vi "swingup_energy_controller.vi"(1 "mu (m/s^2/J)":dbl, 2 "max_u (m/s^2)":dbl=5.0, 3 "alpha_dot (rad/s)":dbl, 4 "alpha_full (rad)":dbl, 5 "E (mJ)":dbl, 6 "Er (mJ)":dbl) -> (0 "u (m/s^2)":dbl)   [LabVIEW 2010]
doc: "Calculates the desired linear acceleration of the pendulum pivot required to swing the pendulum towards the upright position."
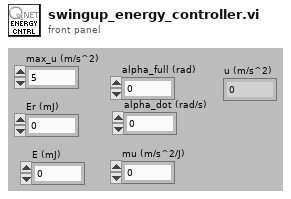
[diagram p1: front panel]
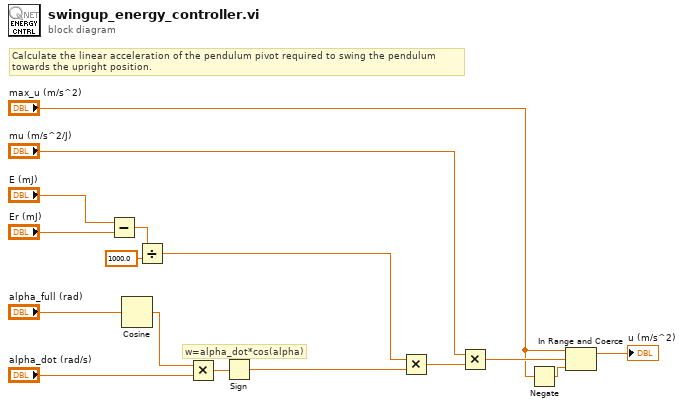
[diagram p0: block diagram]
diagram:
  # "w=alpha_dot*cos(alpha)"
  # "Calculate the linear acceleration of the pendulum pivot required to swing the pendulum towards the upright position."
  n1 = Subtract(x="E (mJ)", y="Er (mJ)") -> (x-y=w2:dbl)
  n2 = Cosine(x="alpha_full (rad)") -> (cos(x)=w16:dbl)
  n3 = Divide(x=w2, y=1000.0) -> (x/y=w1:dbl)
  n4 = Multiply(x=w16, y="alpha_dot (rad/s)") -> (x*y=w14:dbl)
  n5 = Sign(1:w14) -> (0:w13:dbl)
  n6 = Multiply(x=w1, y=w13) -> (x*y=w6:dbl)
  n7 = Multiply(x="mu (m/s^2/J)", y=w6) -> (x*y=w11:dbl)
  n8 = Negate(x="max_u (m/s^2)") -> (-x=w9:dbl)
  n9 = In Range and Coerce(upper limit="max_u (m/s^2)", x=w11, lower limit=w9) -> (coerced(x)=→"u (m/s^2)":dbl)  [unwired: 1 out]
